vi "your step name here.vi"(0 "Setup in":T6={"No.VI"=0, "Category"="", "StepName"="", "Seq setup flattened"="", "Comment"="", "Steps config."=[], "Jump config"=[], "Start"=0.0, "Increment"=0.0, "Name"="Pa", "Unit"="Pa", "Y data"=1, "Y prefix"="", "Y dB ref"=1.0, "Y unit"="", "Repeat State Array"=[]} {"Repeat State Array"."Start" format="%#_5g"; "Y dB ref" format="%.1f"; "Y data" items=["dB", "Lin"]; "Start" format="%#_5g"}, 5 "Data in":T4 {"Z data" items=["dB", "Lin"]; "X data" items=["dB", "Lin"]; "Y data" items=["dB", "Lin"]; "Z dB ref" format="%.1f"; "Z axis" items=["Log", "Lin"]; "X dB ref" format="%.1f"; "X axis" items=["Log", "Lin"]; "Y axis" items=["Log", "Lin"]; "Y dB ref" format="%.1f"; "Curve"."z" format="%.2f"; "Curve"."y" format="%.2f"; "Curve"."x" format="%.2f"}, 7 "Results in":T2 {"Margin" format="%.2f"}, 9 "Seq Setup in":string, 11 "Step name":string, 12 "Hardware in":string, 13 "Calibration in":string) -> (3 "Types Out":string[](array[string]), 4 "Inserted Names Out":string[](array[string]), 6 "Data out":T4 {"Z data" items=["dB", "Lin"]; "X data" items=["dB", "Lin"]; "Y data" items=["dB", "Lin"]; "Z dB ref" format="%.1f"; "Z axis" items=["Log", "Lin"]; "X dB ref" format="%.1f"; "X axis" items=["Log", "Lin"]; "Y axis" items=["Log", "Lin"]; "Y dB ref" format="%.1f"; "Curve"."z" format="%.2f"; "Curve"."y" format="%.2f"; "Curve"."x" format="%.2f"}, 8 "Results out":T2 {"Margin" format="%.2f"}, 10 "Wave out":T1[](array[typedef]) {"Y dB ref" format="%.1f"; "Y axis" items=["Log", "Lin"]; "Y data" items=["dB", "Lin"]; "X data" items=["dB", "Lin"]})   [LabVIEW 2013]
uses:
  CRYCustom and Run Seq.llb/CRYData Cluster Array.ctl
  CRYCustom and Run Seq.llb/CRYData Cluster.ctl
  CRYCustom and Run Seq.llb/CRYResult Cluster Array.ctl
  CRYCustom and Run Seq.llb/CRYResult Cluster.ctl
  CRYCustom and Run Seq.llb/CRYStep.ctl
  CRYCustom and Run Seq.llb/CRYWaveform Cluster.ctl
panel:
  out "example display":string="Motion complete!"
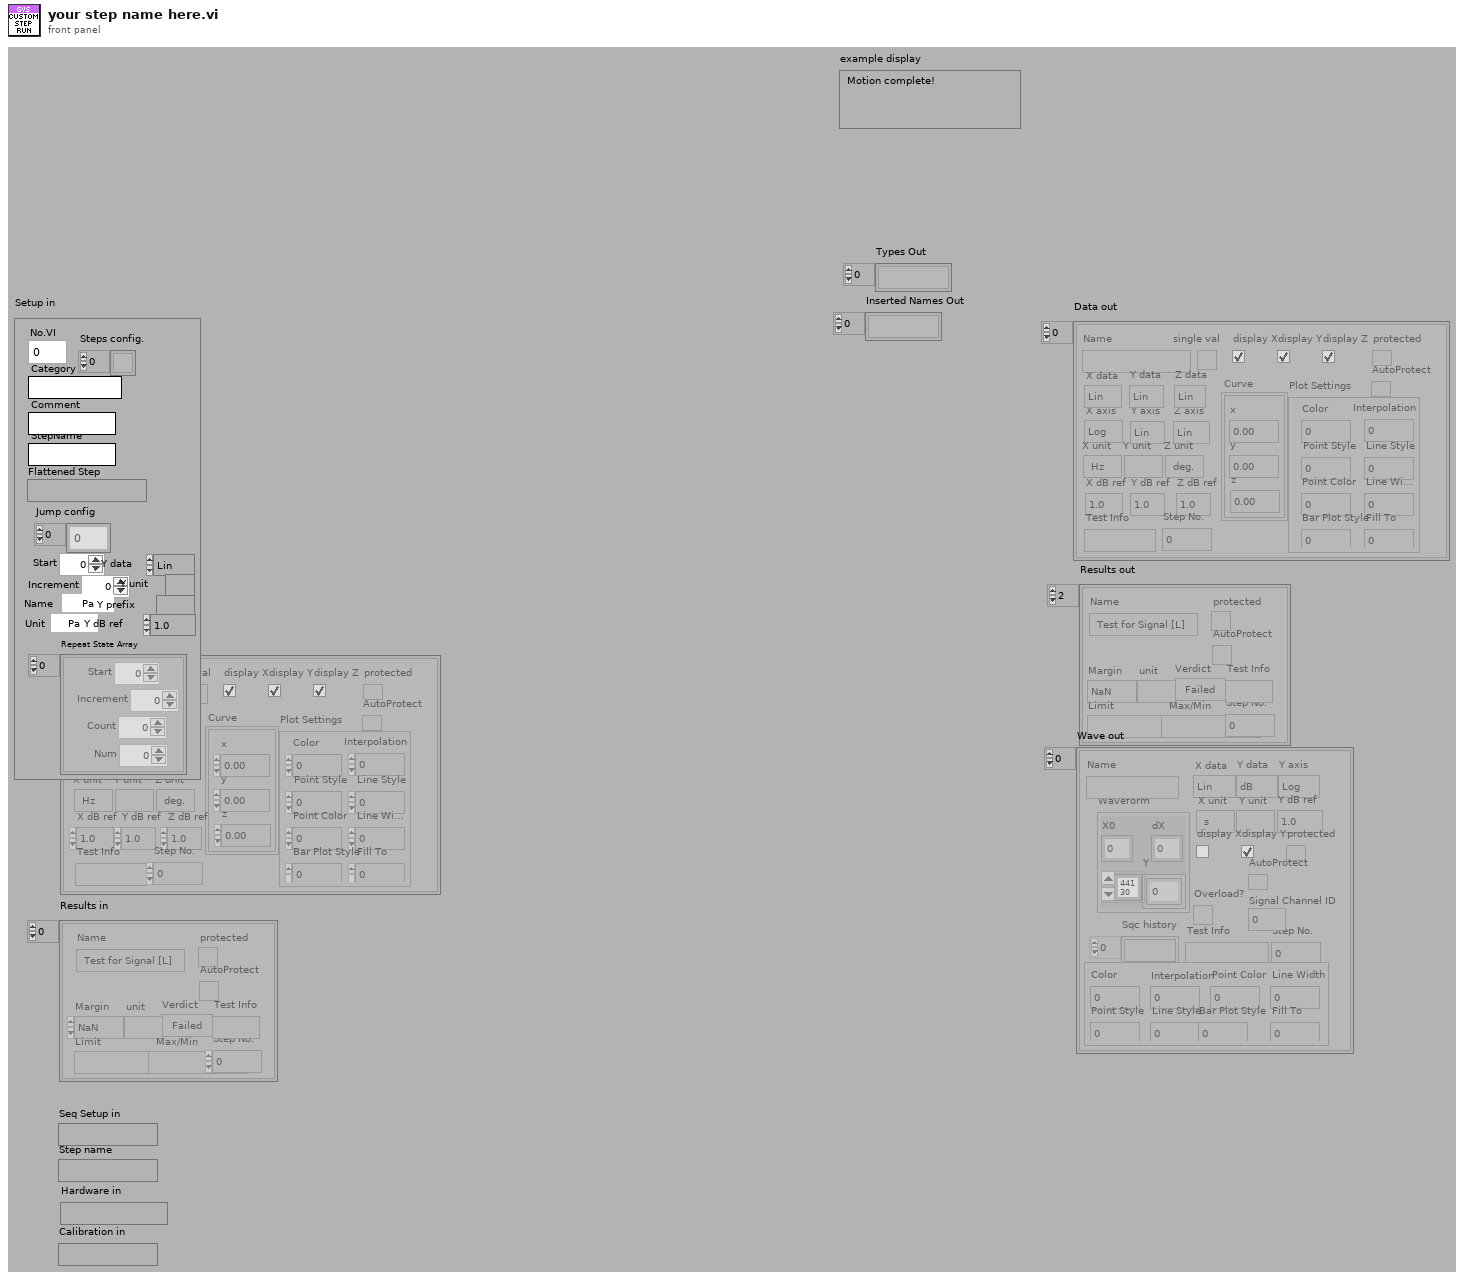
[diagram p1: front panel]
types:
  T1 = typedef "CRYWaveform Cluster.ctl" = cluster{"Waveform":cluster{"X0":dbl, "dX":dbl, "Y":sgl[]}, "X data":u16, "Y data":u16, "Y axis":u16, "X unit":string, "Y unit":string, "Y dB ref":dbl, "display Y":bool, "display X":bool, "Overload?":bool, "Test Info":string, "Step No.":i32, "Name":string, "protected":bool, "Sqc history":string[], "Signal Channel ID":i32, "Plot Settings":cluster{"Color":u32, "Interpolation":u8, "Point Style":u8, "Line Style":u8, "Point Color":u32, "Line Width":u8, "Bar Plot Style":u8, "Fill To":i16}, "AutoProtect":bool}
  T2 = typedef "CRYResult Cluster Array.ctl" = T3[]
  T3 = typedef "CRYResult Cluster.ctl" = cluster{"Name":string, "Margin":dbl, "unit":string, "Verdict":bool, "Limit":string, "Max/Min":string, "protected":bool, "Step No.":i32, "Test Info":string, "AutoProtect":bool}
  T4 = typedef "CRYData Cluster Array.ctl" = T5[]
  T5 = typedef "CRYData Cluster.ctl" = cluster{"Name":string, "Curve":cluster{"x":dbl, "y":dbl, "z":dbl}[], "X data":u16, "Y data":u16, "Z data":u16, "X axis":u16, "Y axis":u16, "Z axis":u16, "X unit":string, "Y unit":string, "Z unit":string, "X dB ref":dbl, "Y dB ref":dbl, "Z dB ref":dbl, "single val":bool, "protected":bool, "display X":bool, "display Y":bool, "display Z":bool, "Test Info":string, "Step No.":i32, "Plot Settings":cluster{"Color":u32, "Interpolation":u8, "Point Style":u8, "Line Style":u8, "Point Color":u32, "Line Width":u8, "Bar Plot Style":u8, "Fill To":i16}, "AutoProtect":bool}
  T6 = typedef "CRYStep.ctl" = cluster{"No.VI":i32, "Category":string, "StepName":string, "Seq setup flattened":string, "Comment":string, "Steps config.":bool[], "Jump config":i32[], "Start":dbl, "Increment":dbl, "Name":string, "Unit":string, "Y data":u16, "Y prefix":string, "Y dB ref":dbl, "Y unit":string, "Repeat State Array":cluster{"Start":dbl, "Increment":dbl, "Count":i32, "Num":i32}[]}
  T7 = cluster{"Parameter A":dbl, "Parameter B":dbl, "Parameter C":dbl}
  T8 = typedef "CRYCustom Cluster.ctl" = cluster{"Help":string, "Flatten Data":string}
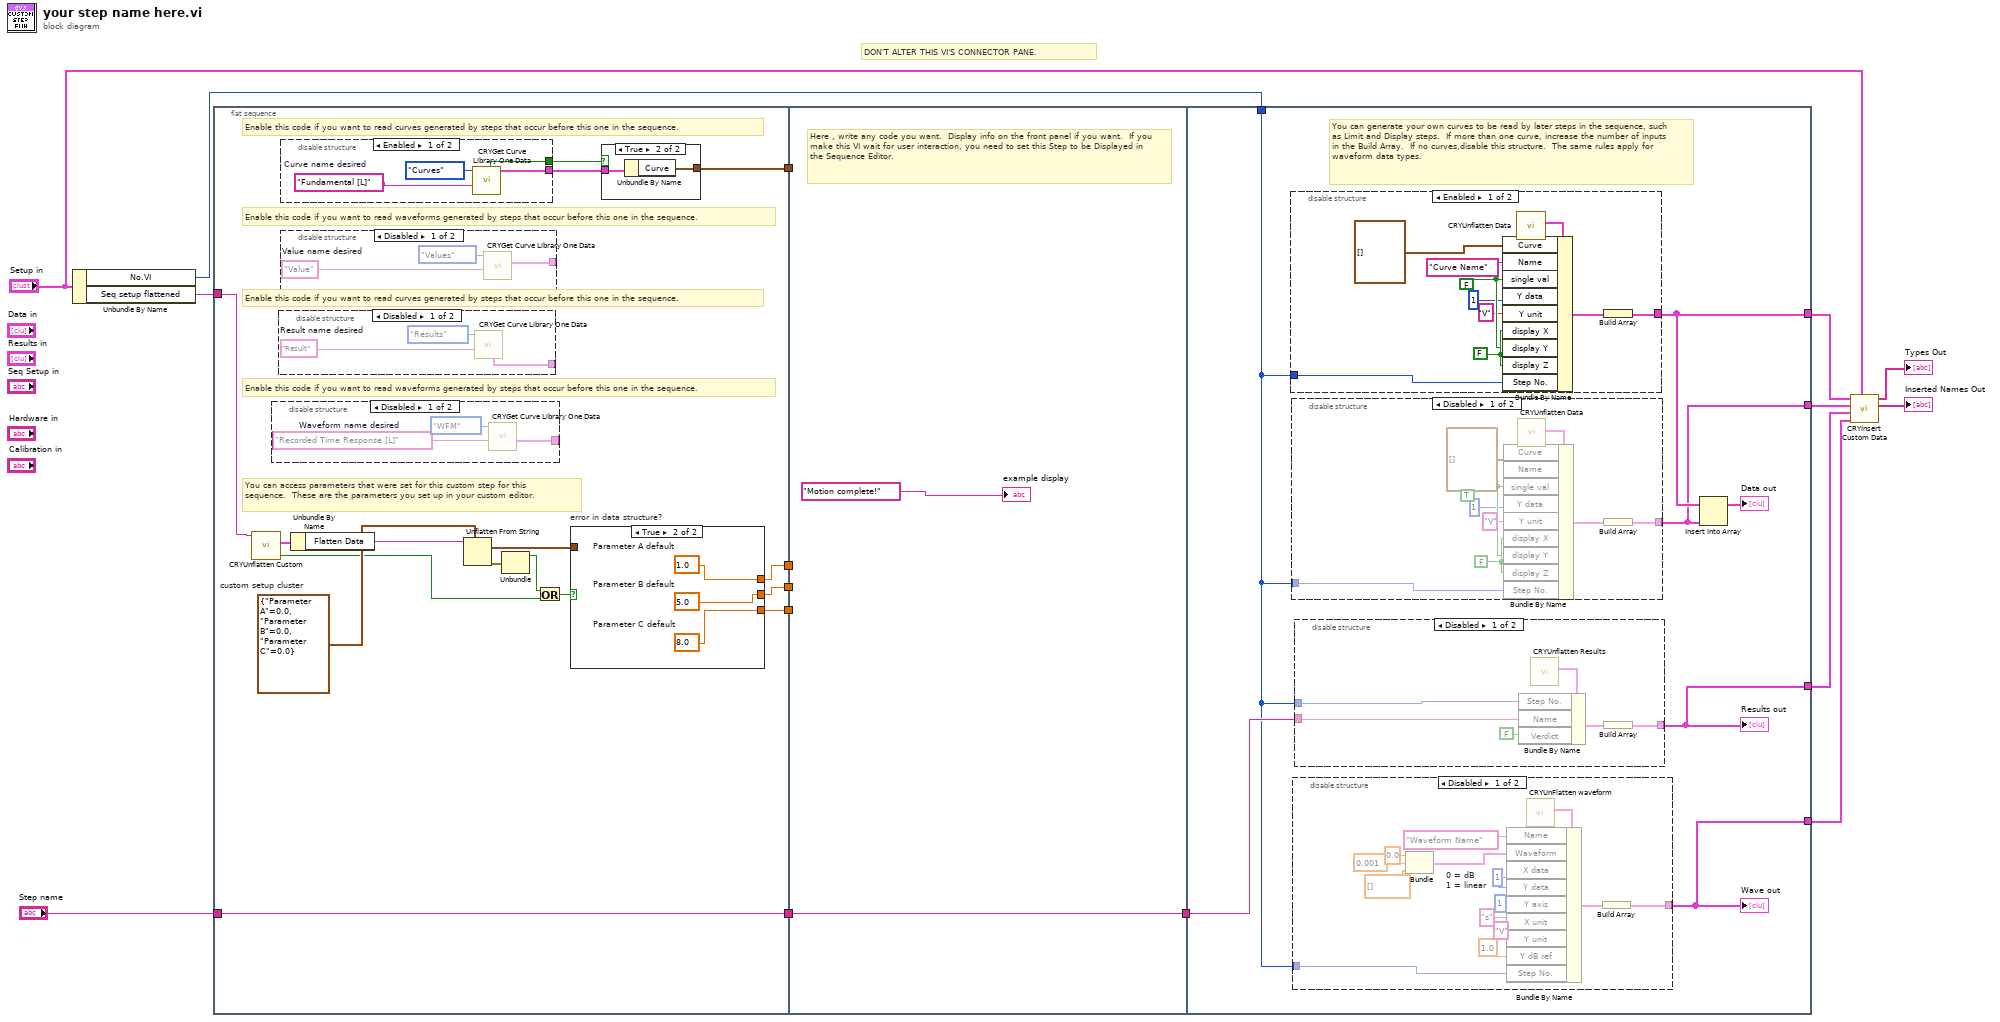
[diagram p0: block diagram]
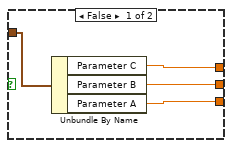
[diagram p7: hidden frame]
diagram:
  # "DON'T ALTER THIS VI'S CONNECTOR PANE."
  n1 = Unbundle By Name("Setup in") -> ("No.VI"=w12:i32, "Seq setup flattened"=w16:string)
  n2 = flat-sequence {
    tunnel: w16 -> [w19]
    tunnel: "Step name" -> [w28]
    tunnel: [w28] -> w14
    tunnel: [w27] -> w4
    tunnel: [w26] -> w3
    tunnel: [w25] -> w2
    tunnel: [w21] -> w1
    tunnel: w14 -> [w56]
    tunnel: [w56] -> w13
    tunnel: w4 -> [_]
    tunnel: w3 -> [_]
    tunnel: w2 -> [_]
    tunnel: w1 -> [_]
    tunnel: w13 -> [w63]
    tunnel: [w62] -> w9
    tunnel: [w58] -> w10
    tunnel: w12 -> [w60]
    tunnel: [w61] -> w8
    tunnel: [w59] -> w11
    frame #0 {
      w24 = T7 {"Parameter A"=0.0, "Parameter B"=0.0, "Parameter C"=0.0}  # custom setup cluster
      # "Enable this code if you want to read waveforms generated by steps that occur before this one in the sequence."
      # "Enable this code if you want to read curves generated by steps that occur before this one in the sequence."
      # "Enable this code if you want to read waveforms generated by steps that occur before this one in the sequence."
      # "Enable this code if you want to read curves generated by steps that occur before this one in the sequence."
      # "You can access parameters that were set for this custom step for this sequence.  These are the parameters you set up in your custom editor."
      n3 = call "CRYUnflatten Custom.vi"("Unflatten Custom"=w19) -> ("Error?"=w18:bool, "Custom"=w20:T8)  [unwired: 8 in, 1 out]
      n4 = disable-structure shown="Disabled" {
        disable-tunnel: [w39 _] -> _
        frame Disabled {
          w38 = "Recorded Time Response [L]"  # Waveform name desired
          n5 = call "CRYGet Curve Library One Data .vi"("Data Name"=w38, "Type"=enum16{"Curves", "Values", "Results", "WFM"}."WFM") -> ("Wave"=w39:T1)  [unwired: 3 in, 6 out]
        }
        frame Enabled {
        }
      }
      n6 = disable-structure shown="Disabled" {
        disable-tunnel: [w35 _] -> _
        frame Disabled {
          w36 = "Result"  # Result name desired
          n7 = call "CRYGet Curve Library One Data .vi"("Data Name"=w36, "Type"=enum16{"Curves", "Values", "Results", "WFM"}."Results") -> ("Result"=w35:T3)  [unwired: 3 in, 6 out]
        }
        frame Enabled {
        }
      }
      n8 = disable-structure shown="Enabled" {
        disable-tunnel: [w42 _] -> w23
        disable-tunnel: [w41 _] -> w22
        frame Enabled {
          w43 = "Fundamental [L]"  # Curve name desired
          n9 = call "CRYGet Curve Library One Data .vi"("Data Name"=w43, "Type"=enum16{"Curves", "Values", "Results", "WFM"}."Curves") -> ("Curve"=w42:T5, "Result"=w41:bool)  [unwired: 3 in, 5 out]
        }
        frame Disabled {
        }
      }
      n10 = disable-structure shown="Disabled" {
        disable-tunnel: [w45 _] -> _
        frame Disabled {
          w46 = "Value"  # Value name desired
          n11 = call "CRYGet Curve Library One Data .vi"("Data Name"=w46, "Type"=enum16{"Curves", "Values", "Results", "WFM"}."Values") -> ("Value"=w45:T5)  [unwired: 3 in, 6 out]
        }
        frame Enabled {
        }
      }
      n12 = Unbundle By Name(w20) -> ("Flatten Data"=w17:string)
      n13 = Unflatten From String(type=w24, binary string=w17) -> (value=w31:T7, error out=w32:errorcluster)  [unwired: 1 in, 3 out]
      n14 = Unbundle(w32) -> ("status"=w29:bool)  [unwired: 2 out]
      n15 = Or(x=w29, y=w18) -> (x .or. y?=w30:bool)
      n16 = case "error in data structure?" shown="True" w30 {
        tunnel: w31 -> [w51 _]
        tunnel: [w50 w54] -> w27
        tunnel: [w49 w53] -> w25
        tunnel: [w48 w52] -> w26
        frame False {
          n17 = Unbundle By Name(w51) -> ("Parameter C"=w50:dbl, "Parameter B"=w49:dbl, "Parameter A"=w48:dbl)
        }
        frame True {
          w52 = 8.0  # Parameter C default
          w53 = 5.0  # Parameter B default
          w54 = 1.0  # Parameter A default
        }
      }
      n18 = case shown="True" w22 {
        tunnel: w23 -> [_ w34]
        tunnel: [_ w33] -> w21
        frame False {
        }
        frame True {
          n19 = Unbundle By Name(w34) -> ("Curve"=w33:cluster{"x":dbl, "y":dbl, "z":dbl}[])
        }
      }
    }
    frame #1 {
      # "Here , write any code you want.  Display info on the front panel if you want.  If you make this VI wait for user interaction, you need to set this Step to be Displayed in the Sequence Editor."
      "example display" <- "Motion complete!" ("example display")
    }
    frame #2 {
      # "You can generate your own curves to be read by later steps in the sequence, such as Limit and Display steps.  If more than one curve, increase the number of inputs in the Build Array.  If no curves,disable this structure.  The same rules apply for waveform data types."
      n20 = disable-structure shown="Enabled" {
        disable-tunnel: w60 -> [w69 _]
        disable-tunnel: [w64 _] -> w59
        frame Enabled {
          w72 = FALSE
          w71 = FALSE
          n21 = call "CRYUnflatten Data.vi"() -> ("Datum"=w73:T5)  [unwired: 9 in, 2 out]
          n22 = Bundle By Name(cluster=w73, "Curve"=cluster{"x":dbl, "y":dbl, "z":dbl}[] [] ("appended array"), "Name"="Curve Name", "single val"=w71, "Y data"=u16 1, "Y unit"="V", "display X"=w72, "display Y"=w71, "display Z"=w72, "Step No."=w69) -> (w65:T5)
          n23 = Build Array(w65) -> (w64:T5[])
        }
        frame Disabled {
        }
      }
      n24 = disable-structure shown="Disabled" {
        disable-tunnel: w60 -> [w78 _]
        disable-tunnel: [w76 _] -> w58
        frame Disabled {
          w81 = FALSE
          w80 = TRUE
          n25 = call "CRYUnflatten Data.vi"() -> ("Datum"=w82:T5)  [unwired: 9 in, 2 out]
          n26 = Bundle By Name(cluster=w82, "Curve"=cluster{"x":dbl, "y":dbl, "z":dbl}[] [], "single val"=w80, "Y data"=u16 1, "Y unit"="V", "display X"=w81, "display Y"=w80, "display Z"=w81, "Step No."=w78) -> (w77:T5)  [unwired: 1 in]
          n27 = Build Array(w77) -> (w76:T5[])
        }
        frame Enabled {
        }
      }
      n28 = disable-structure shown="Disabled" {
        disable-tunnel: [w90 _] -> w61
        disable-tunnel: w60 -> [w89 _]
        frame Disabled {
          w95 = u16 1  # 0 = dB 1 = linear
          n29 = Bundle ("Actual waveform data bundle.\nX0\ndX\n[Y] array")(0.0, 0.001, dbl[] []) -> (w99:cluster{dbl, dbl, dbl[]})  [unwired: 1 out]
          n30 = call "CRYUnFlatten waveform.vi"() -> ("Waveform Cluster"=w100:T1)  [unwired: 9 in, 2 out]
          n31 = Bundle By Name(cluster=w100, "Name"="Waveform Name" ("Bundle Element"), "Waveform"=w99, "X data"=w95, "Y data"=w95, "Y axis"=u16 1, "X unit"="s", "Y unit"="V", "Y dB ref"=1.0, "Step No."=w89) -> (w101:T1)
          n32 = Build Array(w101) -> (w90:T1[])
        }
        frame Enabled {
        }
      }
      "Wave out" <- w61
      n33 = disable-structure shown="Disabled" {
        disable-tunnel: w60 -> [w86 _]
        disable-tunnel: w63 -> [w85 _]
        disable-tunnel: [w84 _] -> w62
        frame Disabled {
          n34 = call "CRYUnflatten Results.vi"() -> ("Result"=w87:T3)  [unwired: 9 in, 2 out]
          n35 = Bundle By Name(cluster=w87, "Step No."=w86, "Name"=w85, "Verdict"=FALSE) -> (w88:T3)
          n36 = Build Array(w88) -> (w84:T3[])
        }
        frame Enabled {
        }
      }
      "Results out" <- w62
      n37 = Insert Into Array(array=w59, new element=w58) -> (→"Data out":T5[])  [unwired: 1 in]
    }
  }
  n38 = call "CRYInsert Custom Data.vi"("Setup in"="Setup in", "Wave"=w8, "Results"=w9, "Values"=w10, "Curves"=w11) -> ("Inserted Names Out"=→"Inserted Names Out":string[], "Types Out"=→"Types Out":string[])  [unwired: 5 in]
